vi "Get Number Of Segments.vi"(8 "error in (no error)":errorcluster, 11 "VISA resource name":refnum<visa-resource-name>) -> (0 "error out":errorcluster, 2 "Number Of Segments":i32, 3 "VISA resource name out":refnum<visa-resource-name>)   [LabVIEW 2015, in "LeCroy Wave Series.lvlib"]
doc: "Get the number of segments which are acquired from device, which is in sequence mode."
uses:
  <instrlib>/LeCroy Wave Series/LeCroy Wave Series.lvlib
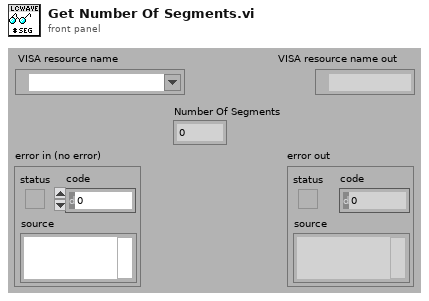
[diagram p1: front panel]
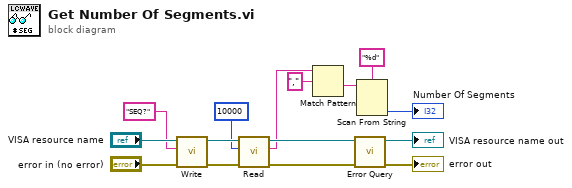
[diagram p0: block diagram]
diagram:
  n1 = call <instrlib>:"Write.vi"("error in (no error)"="error in (no error)", "Write Buffer"="SEQ?", "VISA resource name"="VISA resource name") -> ("error out"=w15:errorcluster, "VISA resource name out"=w14:refnum<visa-resource-name>)  [unwired: 6 in, 1 out]
  n2 = call <instrlib>:"Read.vi"("error in (no error)"=w15, "Byte Count"=u32 10000, "VISA resource name"=w14) -> ("error out"=w8:errorcluster, "Read Buffer"=w5:string, "VISA resource name out"=w9:refnum<visa-resource-name>)  [unwired: 5 in, 1 out]
  n3 = Match Pattern(string=w5, regular expression=",") -> (after substring=w3:string)  [unwired: 1 in, 3 out]
  n4 = call <instrlib>:"Error Query.vi"("error in (no error)"=w8, "VISA resource name"=w9) -> ("error out"=→"error out":errorcluster, "VISA resource name out"=→"VISA resource name out":refnum<visa-resource-name>)  [unwired: 6 in, 2 out]
  n5 = Scan From String(format string="%d", input string=w3) -> (output 1=→"Number Of Segments":i32)  [unwired: 3 in, 3 out]
